vi "Write.vi"(8 "Check Busy Flag?":bool=TRUE, 10 "Data":u8, 11 "Register Select":bool) -> ()   [LabVIEW 2019, in "HD44780.lvlib"]
uses:
  HD44780.lvlib
  <vilib>/rvi/eio/common/nirviEmuTemplateMethod_errors.vi
  <vilib>/eio/EIONode/EIONode.xnode
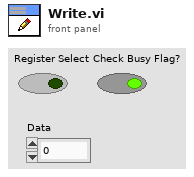
[diagram p1: front panel]
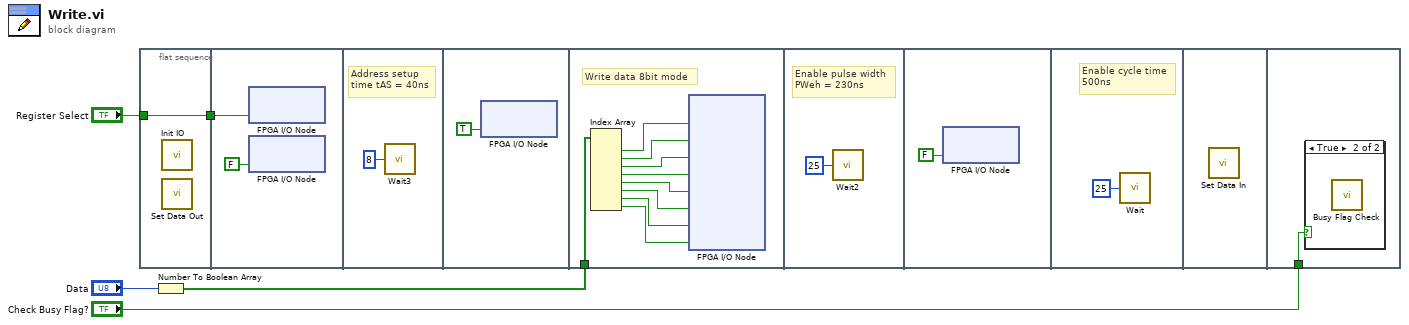
[diagram p0: block diagram]
diagram:
  n1 = flat-sequence {
    tunnel: "Register Select" -> [w6]
    tunnel: [w6] -> w2
    tunnel: w2 -> [w8]
    tunnel: w3 -> [w11]
    tunnel: "Check Busy Flag?" -> [w23]
    frame #0 {
      n2 = call "Init IO.vi"() -> ()  [unwired: 12 in]
      n3 = call "Set Data Out.vi"() -> ()  [unwired: 12 in]
    }
    frame #1 {
      n4 = xnode "FPGA I/O Node"("RS"=w8) -> ()  [unwired: 1 in, 1 out]
      n5 = xnode "FPGA I/O Node"("RW"=FALSE) -> ()  [unwired: 1 in, 1 out]
    }
    frame #2 {
      # "Address setup\ntime tAS = 40ns"
      n6 = call "Wait3"("Count(Ticks)"=u8 8 ("Count(uSec)")) -> ()  [unwired: 1 out]
    }
    frame #3 {
      n7 = xnode "FPGA I/O Node"("E"=TRUE) -> ()  [unwired: 1 in, 1 out]
    }
    frame #4 {
      # "Write data 8bit mode"
      n8 = Index Array(array=w11) -> (element #1=w12:bool, element #2=w13:bool, element #3=w14:bool, element #4=w15:bool, element #5=w16:bool, element #6=w17:bool, element #7=w18:bool, element #8=w19:bool)  [unwired: 8 in]
      n9 = xnode "FPGA I/O Node"("DB0"=w12, "DB1"=w13, "DB2"=w14, "DB3"=w15, "DB4"=w16, "DB5"=w17, "DB6"=w18, "DB7"=w19) -> ()  [unwired: 8 in, 8 out]
    }
    frame #5 {
      # "Enable pulse width\nPWeh = 230ns"
      n10 = call "Wait2"("Count(Ticks)"=u8 25 ("Count(uSec)")) -> ()  [unwired: 1 out]
    }
    frame #6 {
      n11 = xnode "FPGA I/O Node"("E"=FALSE) -> ()  [unwired: 1 in, 1 out]
    }
    frame #7 {
      # "Enable cycle time\n500ns"
      n12 = call "Wait"("Count(Ticks)"=u8 25 ("Count(uSec)")) -> ()  [unwired: 1 out]
    }
    frame #8 {
      n13 = call "Set Data In.vi"() -> ()  [unwired: 12 in]
    }
    frame #9 {
      n14 = case shown="True" w23 {
        frame False {
        }
        frame True {
          n15 = call "Busy Flag Check.vi"() -> ()  [unwired: 12 in]
        }
      }
    }
  }
  n16 = Number To Boolean Array(number="Data") -> (Boolean array=w3:bool[])
